vi "Lian_Iteration_Counter.vi"() -> ()   [LabVIEW 2020]
panel:
  in  "?":bool
  out "Required Iterations":i32
  out "Random  Number":dbl
  # "Iteration Counter"
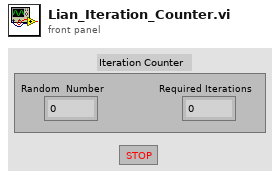
[diagram p1: front panel]
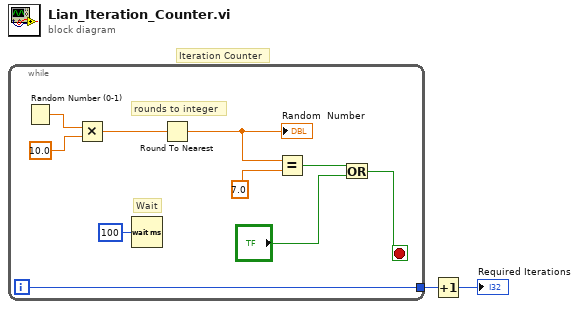
[diagram p0: block diagram]
diagram:
  # "Iteration Counter"
  n1 = while {
    tunnel: [w3] -> w2
    i -> [w3]
    stop <- w5 stop-if-true
    # "Wait"
    # "rounds to integer"
    n2 = Random Number (0-1)() -> (number: 0 to 1=w9:dbl)
    n3 = Multiply(x=w9, y=10.0) -> (x*y=w7:dbl)
    n4 = Wait (ms)(milliseconds to wait=u32 100) -> ()  [unwired: 1 out]
    n5 = Round To Nearest(number=w7) -> (nearest integer value=w12:dbl)
    "Random  Number" <- w12
    n6 = Equal?(x=w12, y=7.0) -> (x = y?=w6:bool)
    n7 = Or(x=w6, y="?") -> (x .or. y?=w5:bool)
  }
  n8 = Increment(x=w2) -> (x+1=→"Required Iterations":i32)
